vi "chart set style.vi"(8 "error in (no error)":errorcluster, 10 "style_id":T1 items=["Style_1", "Style_2", "Style_3", "Style_4", "Style_5", "Style_6", "Style_7", "Style_8", "Style_9", "Style_10", "Style_11", "Style_12", "Style_13", "Style_14", "Style_15", "Style_16", "Style_17", "Style_18", "Style_19", "Style_20", "Style_21", "Style_22", "Style_23", "Style_24", "Style_25", "Style_26", "Style_27", "Style_28", "Style_29", "Style_30", "Style_31", "Style_32", "Style_33", "Style_34", "Style_35", "Style_36", "Style_37", "Style_38", "Style_39", "Style_40", "Style_41", "Style_42", "Style_43", "Style_44", "Style_45", "Style_46", "Style_47", "Style_48"], 11 "chart":u32) -> (0 "error out":errorcluster)   [LabVIEW 8.6]
doc: "void chart_set_style(lxw_chart chart, uint8_t style_id);"
uses:
  pending_lvxlsxwriter/xlsxwriter.dll
  Controls/style_id.ctl
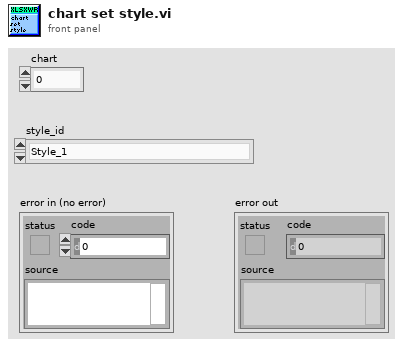
[diagram p1: front panel]
types:
  T1 = typedef "style_id.ctl" = u16
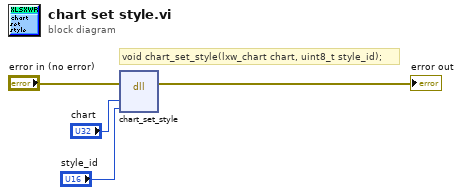
[diagram p0: block diagram]
diagram:
  # "void chart_set_style(lxw_chart chart, uint8_t style_id);"
  n1 = dll-call lib="C:/Users/WDAGUtilityAccount/Desktop/pending_lvxlsxwriter/xlsxwriter.*" fn="chart_set_style"(error in="error in (no error)", "chart"="chart", "style_id"="style_id") -> (error out=→"error out":errorcluster)  [unwired: 5 in, 1 out]
